vi "Remove FIFO Publisher Command.vi"(8 "error in (no error)":errorcluster, 9 "Timeout (ms)":u32=1000, 10 "Publisher Name":string, 11 "CIFChannelMng in":refnum<class "CIFChannelMng.lvclass">) -> (0 "error out":errorcluster, 1 "Timeout":bool, 2 "FIFO Publisher":T1, 3 "CIFChannelMng out":refnum<class "CIFChannelMng.lvclass">)   [LabVIEW 2021, in "CIFChannelMng.lvclass"]
uses:
  CIFChannelMng.lvclass
  OOB/OOB_Tx/Typedef/FIFO Publisher Return.ctl
  CIFChannelMng.lvclass/CIFChannelMng.ctl
  <vilib>/CIF Foundation/CIF Out of Band Commands/CIFOutOfBand.lvclass/CIFOutOfBand.ctl
  OOB/OOB_Tx/Receive/Check for OOB Commands.vi
  OOB/OOB_Tx/Receive/Read Channel List.vi
  OOB/OOB_Tx/Receive/Read New FIFO Publisher.vi
  <vilib>/CIF Foundation/CIF Out of Band Commands/Accessors/Read Local OOB Data.vi
  <vilib>/CIF Foundation/CIF Out of Band Commands/Queue Command.vi
  <vilib>/CIF Foundation/CIF Out of Band Commands/Utilities/Command to Bitwise Command.vi
  <vilib>/CIF Foundation/CIF Out of Band Commands/Read Commands.vi
  OOB/OOB_Tx/Private/Command Settings.vi
  OOB/OOB_Tx/Private/Read Payload.vi
  OOB/OOB_Rx/ChanMngOOB_Rx.lvclass
  C:/Program Files/National Instruments/LabVIEW 2021/vi.lib/CIF Foundation/CIF Out of Band Commands/CIFOutOfBand.lvclass
  OOB/OOB_Tx/ChnMngOOB_Tx.lvclass
  <vilib>/CIF Foundation/CIF Out of Band Commands/CIFOutOfBand.lvclass
  D:/dev/CIF-LVCore/src/Channels/CIFChannelMng/OOB/OOB_Rx/ChanMngOOB_Rx.lvclass
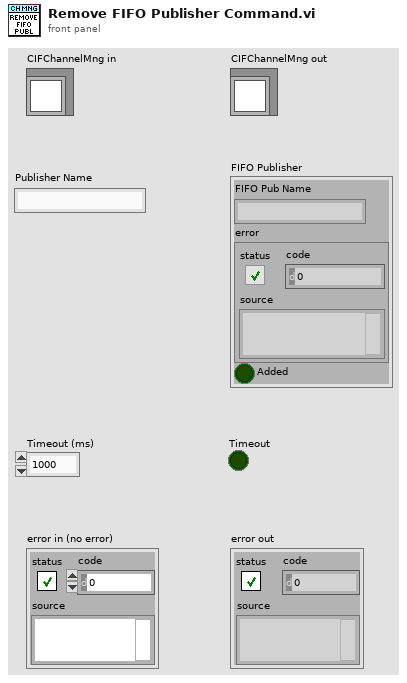
[diagram p1: front panel]
types:
  T1 = typedef "ChnMngOOB_Tx.lvclass/FIFO Publisher Return.ctl" = cluster{"FIFO Pub Name":string, "error":errorcluster, "Added":bool}
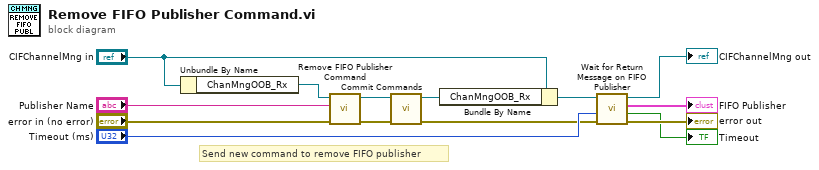
[diagram p0: block diagram]
diagram:
  # "Send new command to remove FIFO publisher"
  n1 = Unbundle By Name("CIFChannelMng in") -> ("ChanMngOOB_Rx"=w7:refnum<class "ChanMngOOB_Rx.lvclass">)
  n2 = call "Remove FIFO Publisher Command.vi"("error in"="error in (no error)", "Publisher Name"="Publisher Name", "ChanMngOOB_Rx in"=w7) -> ("error out"=w2:errorcluster, "ChanMngOOB_Rx out"=w4:refnum<class "ChanMngOOB_Rx.lvclass">)  [unwired: 7 in]
  n3 = call <vilib>:"Commit Commands.vi"("error in"=w2, "OOB in"=w4) -> ("error out"=w1:errorcluster, "OOB out"=w3:refnum<class "ChanMngOOB_Rx.lvclass">)  [unwired: 8 in]
  n4 = Bundle By Name(cluster="CIFChannelMng in", "ChanMngOOB_Rx"=w3) -> (w13:refnum<class "CIFChannelMng.lvclass">)
  n5 = call "Wait for Return Message on FIFO Publisher.vi"("error in (no error)"=w1, "Timeout (ms)"="Timeout (ms)", "CIFChannelMng in"=w13) -> ("error out"=→"error out":errorcluster, "Timeout"=→"Timeout":bool, "FIFO Publisher"=→"FIFO Publisher":T1, "CIFChannelMng out"=→"CIFChannelMng out":refnum<class "CIFChannelMng.lvclass">)  [unwired: 5 in]
